vi "trash_Core Read U8 FIFO External Payload.vi"(8 "error in (no error)":errorcluster, 9 "Timeout (ms)":i32, 11 "CIFFIFO in":refnum<class "CIF_CIPC_Fifo_U8.lvclass">) -> (0 "error out":errorcluster, 1 "timed out?":bool, 3 "CIFFIFO out":refnum<class "CIF_CIPC_Fifo_U8.lvclass">)   [LabVIEW 2021]
doc: "Return the full payload bytes, including the encoded header. This is intended for advanced applications where the full buffer will be passed externally."
uses:
  CIF_CIPC_Fifo_U8.lvclass
  D:/dev/Packages/CIF_Channels_Core/src/CIFChannels/CIFChannels.lvclass
  D:/dev/Packages/CIF_Channels_Core/src/CIPC_Channels/CIF_CIPC_Chan/CIF_CIPC_Chn.lvclass
  CIFChannels/Typedef/Channel State.ctl
  CIFChannels/Typedef/Direction.ctl
  CIFChannels/CIFChannels.lvclass/CIFChannels.ctl
  <vilib>/CIF Foundation/CIF CIPC/TypeDefs/Data Element Details.ctl
  <vilib>/CIF Foundation/CIF CIPC/TypeDefs/Read Configuration.ctl
  <vilib>/CIF Foundation/CIF CIPC/TypeDefs/Read Position.ctl
  CIF_CIPC_Chan/CIF_CIPC_Chn.lvclass/CIF_CIPC_Chn.ctl
  CIF_CIPC_Fifo_U8.lvclass/CIF_CIPC_Fifo_U8.ctl
  <vilib>/CIF Foundation/CIF Utilities/Statistics/I64/Stats_I64_CIF_U.lvclass/Stats_I64_CIF_U.ctl
  e703c505-0034-46a9-8989-21c0de27793f.vi
  768488f4-e6df-4560-a449-a64b33b49031.vi
  CIFChannels/Accessors/Read Channel State.vi
  CIFChannels/Accessors/Read Direction.vi
  <vilib>/CIF Foundation/CIF Utilities/DataTypes/Flatten Unflatten/Unflatten U64.vi
  <vilib>/CIF Foundation/CIF Utilities/DataTypes/Flatten Unflatten/Unflatten I64.vi
  ChannelCommon/Utilities/Add Error.vi
  CIF_CIPC_Chan/Accessors/Read CIPC Channel.vi
  Read Wrapper for Backpressure Support.vi/b5615cf0-cd7f-4476-b9a9-d6ef7628cc3b.vi
  CIF_CIPC_Chan/Accessors/Read Buffer Configuration.vi
  Read Wrapper for Backpressure Support.vi/6248fc70-cc83-4025-b778-a3221b95feac.vi
  CIFChannels/Accessors/Read FIFO Backpressure.vi
  <vilib>/CIF Foundation/CIF Utilities/Statistics/I64/X1 minus X0.vi
  <vilib>/CIF Foundation/CIF Utilities/Time/System Time/Get System Time.vi
  <vilib>/CIF Foundation/CIF CIPC/SubVIs/Wait For N Elements Available.vi
  <vilib>/CIF Foundation/CIF CIPC/SubVIs/Get Element Read Position.vi
  <vilib>/CIF Foundation/CIF CIPC/SubVIs/Check Error.vi
  <vilib>/CIF Foundation/CIF CIPC/SubVIs/Get dll Path.vi
  <vilib>/CIF Foundation/CIF CIPC/SubVIs/Set Element Read Position.vi
  Read Wrapper for Backpressure Support.vi/6248fc70-cc83-4025-b778-a3221b95feac.vi/331f6ecb-7ec4-4931-b93d-4fbd8d66a851.vi
  Read Wrapper for Backpressure Support.vi/6248fc70-cc83-4025-b778-a3221b95feac.vi/5ce0d4cf-f921-42ba-b14c-c90f7f7611e4.vi
  <vilib>/CIF Foundation/CIF Utilities/Statistics/I64/X1 minus X0.vi/dfabcf33-0dbc-4041-80a5-3dc0c86d2989.vi
  <vilib>/CIF Foundation/CIF Utilities/Time/System Time/LabVIEW Time to TAI Time.vi
  <vilib>/CIF Foundation/CIF CIPC/SubVIs/Notify Of New Write.vi
  <vilib>/CIF Foundation/CIF CIPC/SubVIs/Get Element Write Position.vi
  <vilib>/CIF Foundation/CIF Utilities/Statistics/I64/X1 minus X0.vi/dfabcf33-0dbc-4041-80a5-3dc0c86d2989.vi/9eb60a9a-770f-4d2d-8b3f-8465c267ecc9.vi
  <vilib>/CIF Foundation/CIF CIPC/SubVIs/Check Error Core.vi
  <vilib>/CIF Foundation/CIF CIPC/SubVIs/Get Element Info Variant.vi
  ChannelCommon/Utilities/Add Error Core.vi
  CIFChannels/CIFChannels.lvclass
  ChannelCommon/ChannelCommon.lvlib
  <vilib>/CIF Foundation/CIF CIPC/CIF_NI_CIPC.lvlib
  D:/dev/Packages/CIF_Channels_Core/src/CIPC_Channels/FIFO_U8/CIF_CIPC_Fifo_U8.lvclass
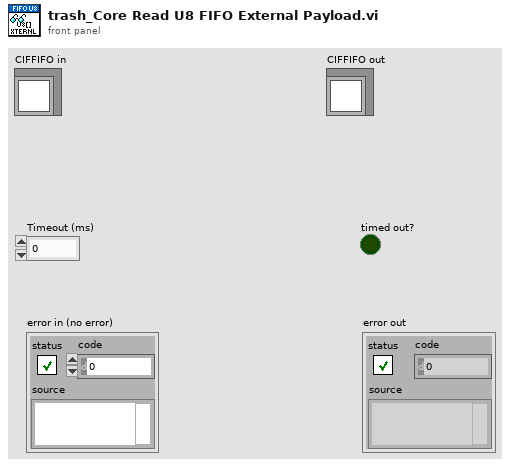
[diagram p1: front panel]
types:
  T1 = typedef "CIFChannels.lvclass/Channel State.ctl" = enum8{"Creating", "Disconnected", "Connecting", "Connected", "Destroyed"}
  T2 = typedef "CIFChannels.lvclass/Direction.ctl" = enum8{"Publisher", "Subscriber"}
  T3 = typedef "CIF_NI_CIPC.lvlib/Data Element Details.ctl" = cluster{"Bytes to Read":u32, "Element Offset":u32}
  T4 = typedef "CIF_NI_CIPC.lvlib/Read Configuration.ctl" = cluster{"Read Position":T5, "Element Offset":i32, "Prepend Array Size":bool, "Get Read Position":bool}
  T5 = typedef "CIF_NI_CIPC.lvlib/Read Position.ctl" = enum8{"Next", "Newest", "Oldest", "Next Available", "Absolute"}
  T6 = typedef "ChannelCommon.lvlib/FIFO Header.ctl" = cluster{"Length":u64, "T0":i64, "T_Out":i64, "T_Tx":i64, "Ctr":u64, "ClockID":u8}
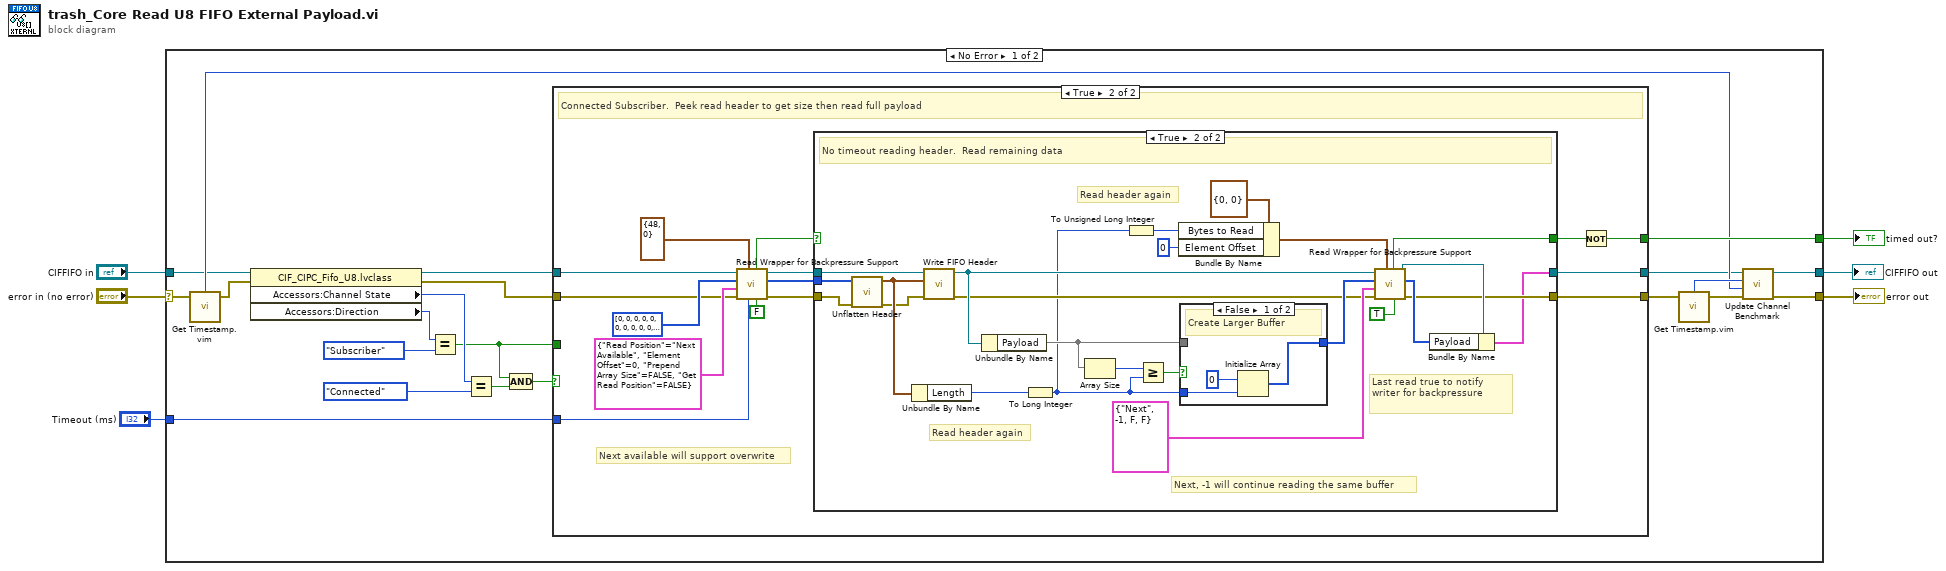
[diagram p0: block diagram]
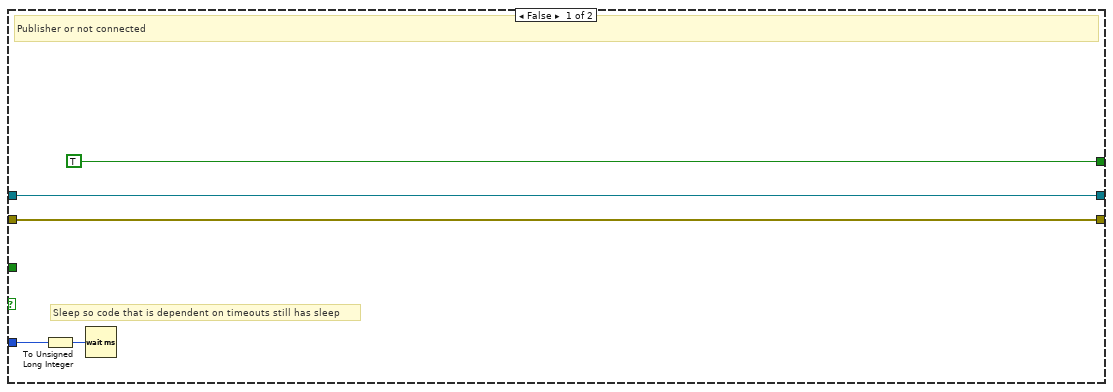
[diagram p2: hidden frame]
diagram:
  n1 = case shown="No Error" "error in (no error)" {
    selector: "error in (no error)" -> [w9 w80]
    tunnel: [w15 w80] -> w1
    tunnel: [w16 w79] -> w2
    tunnel: "CIFFIFO in" -> [w8 w79]
    tunnel: [w27 _] -> w3
    tunnel: "Timeout (ms)" -> [w17 _]
    frame No Error {
      n2 = call "Get Timestamp.vim"("Anything in"=w9) -> ("Time (ns)"=w13:i64, "Anything out"=w7:errorcluster)  [unwired: 2 in]
      n3 = property class="CIF_CIPC_Fifo_U8.lvclass"(reference=w8, error in=w7) -> (reference out=w26:refnum<class "CIF_CIPC_Fifo_U8.lvclass">, error out=w25:errorcluster, "Accessors:Channel State"=w22:T1, "Accessors:Direction"=w24:T2)
      n4 = Equal?(x=w24, y=Direction."Subscriber") -> (x = y?=w18:bool)
      n5 = Equal?(x=w22, y=Channel_State."Connected") -> (x = y?=w20:bool)
      n6 = Compound Arithmetic op=AND(w18, w20) -> (w19:bool)
      n7 = case shown="True" w19 {
        tunnel: [TRUE ("timeout out") w44] -> w27
        tunnel: w25 -> [w31 w35]
        tunnel: w26 -> [w32 w34]
        tunnel: w18 -> [_ _]
        tunnel: [w32 w47] -> w11
        tunnel: [w31 w46] -> w10
        tunnel: w17 -> [w29 w38]
        frame False {
          # "Sleep so code that is dependent on timeouts still has sleep"
          # "Publisher or not connected"
          n8 = To Unsigned Long Integer(number=w29) -> (unsigned 32bit integer=w28:u32)
          n9 = Wait (ms)(milliseconds to wait=w28) -> ()  [unwired: 1 out]
        }
        frame True {
          # "Next available will support overwrite"
          # "Connected Subscriber.  Peek read header to get size then read full payload"
          n10 = call "Read Wrapper for Backpressure Support.vi"("Last Read"=FALSE, "Timeout (ms)"=w38, "Data Element"=T3 {"Bytes to Read"=48, "Element Offset"=0}, "error in (no error)"=w35, "Read Configuration"=T4 {"Read Position"=enum."Next Available", "Element Offset"=0, "Prepend Array Size"=FALSE, "Get Read Position"=FALSE}, "Data in"=u8[] [0, 0, 0, 0, 0, 0, 0, 0, 0, 0, 0, 0, 0, 0, 0, 0, 0, 0, 0, 0, 0, 0, 0, 0, 0, 0, 0, 0, 0, 0, 0, 0, 0, 0, 0, 0, 0, 0, 0, 0, 0, 0, 0, 0, 0, 0, 0, 0] ("U8 Array in"), "CIF_CIPC_Fifo_U8 in"=w34) -> ("error out"=w37:errorcluster, "Data out"=w36:u8[], "CIF_CIPC_Fifo_U8 out"=w43:refnum<class "CIF_CIPC_Fifo_U8.lvclass">, "Success"=w41:bool)  [unwired: 1 out]
          n11 = case shown="True" w41 {
            selector: w41 -> [w48 _]
            tunnel: w43 -> [w50 w61]
            tunnel: w37 -> [w49 w74]
            tunnel: w36 -> [_ w73]
            tunnel: [w49 w57] -> w46
            tunnel: [w50 w56] -> w47
            tunnel: [w48 w54] -> w45
            frame False {
              # "Timeout reading header"
            }
            frame True {
              # "Read header again"
              # "Last read true to notify writer for backpressure"
              # "Read header again"
              # "Next, -1 will continue reading the same buffer"
              # "No timeout reading header.  Read remaining data"
              n12 = call "Unflatten Header.vi"("error in (no error)"=w74, "Flattened Data in"=w73) -> ("error out"=w59:errorcluster, "Header out"=w60:T6)  [unwired: 7 in, 1 out]
              n13 = Unbundle By Name(w60) -> ("Length"=w51:u64)
              n14 = call "Write FIFO Header.vi"("error in (no error)"=w59, "Header"=w60, "CIFChannels in"=w61) -> ("error out"=w55:errorcluster, "CIFChannels out"=w58:refnum<class "CIF_CIPC_Fifo_U8.lvclass">)  [unwired: 7 in]
              n15 = Unbundle By Name(w58) -> ("Payload"=w70)
              n16 = To Long Integer(number=w51) -> (32bit integer=w53:i32)
              n17 = Array Size(array=w70) -> (size(s)=w71:i32)
              n18 = To Unsigned Long Integer(number=w53) -> (unsigned 32bit integer=w69:u32)
              n19 = Greater Or Equal?(x=w71, y=w53) -> (x >= y?=w72:bool)
              n20 = Bundle By Name(cluster=T3 {"Bytes to Read"=0, "Element Offset"=0} ("Data Element"), "Bytes to Read"=w69, "Element Offset"=u32 0) -> (w62:T3)
              n21 = case shown="False" w72 {
                tunnel: w70 -> [_ w78]
                tunnel: [w77 w78] -> w66
                tunnel: w53 -> [w75 _]
                frame False {
                  # "Create Larger Buffer"
                  n22 = Initialize Array(u8 0, w75) -> (w77:u8[])
                }
                frame True {
                  # "Reuse buffer"
                }
              }
              n23 = call "Read Wrapper for Backpressure Support.vi"("Last Read"=TRUE, "Data Element"=w62, "error in (no error)"=w55, "Read Configuration"=T4 {"Read Position"=enum."Next", "Element Offset"=-1, "Prepend Array Size"=FALSE, "Get Read Position"=FALSE}, "Data in"=w66, "CIF_CIPC_Fifo_U8 in"=w58) -> ("error out"=w57:errorcluster, "Data out"=w64:u8[], "CIF_CIPC_Fifo_U8 out"=w63:refnum<class "CIF_CIPC_Fifo_U8.lvclass">, "Success"=w54:bool)  [unwired: 1 in, 1 out]
              n24 = Bundle By Name(cluster=w63, "Payload"=w64) -> (w56:cluster{})
            }
          }
          n25 = Not(x=w45) -> (.not. x?=w44:bool)
        }
      }
      n26 = call "Get Timestamp.vim"("Anything in"=w10) -> ("Time (ns)"=w14:i64, "Anything out"=w12:errorcluster)  [unwired: 2 in]
      n27 = call "Update Channel Benchmark.vi"("error in (no error)"=w12, "X0"=w13, "X1"=w14, "CIFChannels in"=w11) -> ("error out"=w15:errorcluster, "CIFChannels out"=w16:refnum<class "CIF_CIPC_Fifo_U8.lvclass">)  [unwired: 6 in]
    }
    frame Error {
    }
  }
  "error out" <- w1
  "timed out?" <- w3
  "CIFFIFO out" <- w2
